vi "Get Error Info.vi"(11 "Application Error in":refnum<class "Application Error.lvclass">) -> (3 "Application Error out":refnum<class "Application Error.lvclass">, 4 "Time Stamp":timestamp, 5 "Error Name":string, 6 "Error Source":string, 7 "Error Scope":string)   [LabVIEW 2016, in "Stream Error.lvlib" / "Application Error.lvclass"]
doc: "--\nCopyright © 2017 Composed SystemsI All rights reserved.\n\nAuthor: Jon McBee <jon.mcbee@composed.io>\n\nThis library is provided \"AS IS\" ,WITHOUT WARRANTIES OR\nCONDITIONS OF ANY KIND, either express or implied.\n\nComposed Systems -- composed.io\n\nStream 0.0.1.1\nJon McBee - Composed Systems\nCopyright (c) 2017, Composed Systems"
uses:
  <userlib>/Composed Systems/Stream/Error/Classes/Application Error/Application Error.lvclass
  <userlib>/Composed Systems/Stream/Error/Classes/Error Interface/Error Interface.lvclass
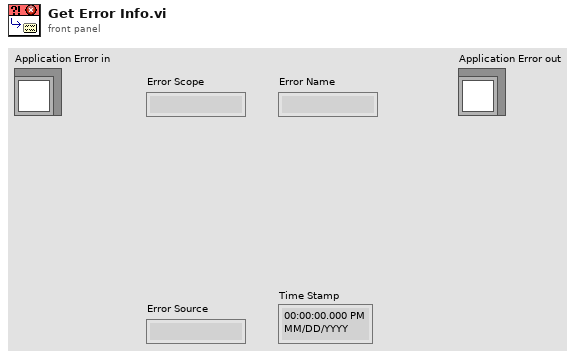
[diagram p1: front panel]
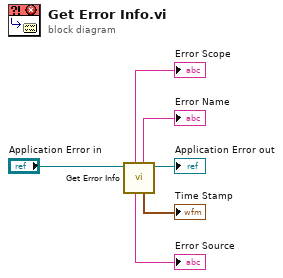
[diagram p0: block diagram]
diagram:
  n1 = call-parent "Get Error Info.vi"("Error Interface in"="Application Error in") -> ("Error Interface out"=→"Application Error out":refnum<class "Application Error.lvclass">, "Time Stamp"=→"Time Stamp":timestamp, "Error Name"=→"Error Name":string, "Error Source"=→"Error Source":string, "Error Scope"=→"Error Scope":string)  [unwired: 6 in]
